vi "Update Step UI Values.vi"(9 "Array":string[][](array[string]), 10 "State cluster":T1, 11 "ListBox in":refnum<vi>) -> (2 "index of element":i32, 3 "Sequence #":i32)   [LabVIEW 2015, in "Sequencer Module tests.lvlib"]
uses:
  module/execution/Sequencer State Cluster.ctl
  module/execution/Sequencer State Enum.ctl
  classes/Step/Execution/StepState.ctl
  classes/Step/Execution/Step Status.ctl
  classes/Step/Execution/Step Flow Control.ctl
  Sequencer Module tests.lvlib
  module/execution/Sequencer Module runtime.lvclass
  classes/Step/Execution/Step.lvclass
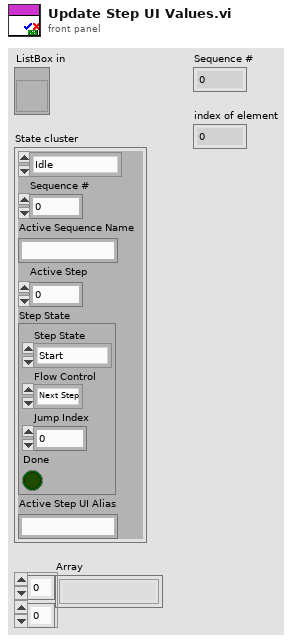
[diagram p1: front panel]
types:
  T1 = typedef "Sequencer Module runtime.lvclass/Sequencer State Cluster.ctl" = cluster{"Sequencer State":T2, "Sequence #":i32, "Active Sequence Name":string, "Active Step":i32, "Step State":T3, "Active Step UI Alias":string}
  T2 = typedef "Sequencer Module runtime.lvclass/Sequencer State Enum.ctl" = enum16{"Idle", "Paused", "Start Sequence", "Run Sequence", "CleanUp Sequence", "Generate Report"}
  T3 = typedef "Step.lvclass/StepState.ctl" = cluster{"Step State":T4, "Flow Control":T5, "Jump Index":i32, "Done":bool}
  T4 = typedef "Step.lvclass/Step Status.ctl" = enum16{"Start", "Passed", "Failed", "Error", "Done", "Terminated", "Skipped", "Running"}
  T5 = typedef "Step.lvclass/Step Flow Control.ctl" = enum16{"Next Step", "Jump"}
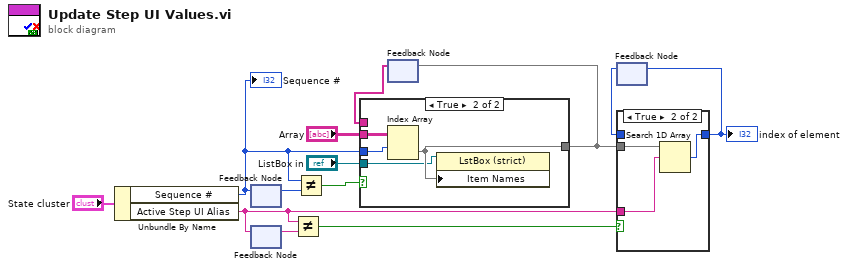
[diagram p0: block diagram]
diagram:
  n1 = Unbundle By Name("State cluster") -> ("Sequence #"=w6:i32, "Active Step UI Alias"=w11:string)
  "Sequence #" <- w6
  n2 = feedback #1() -> (w3:i32)  [unwired: 1 in]
  n3 = feedback-in #1(w6) -> ()
  n4 = feedback #2() -> (w8:string)  [unwired: 1 in]
  n5 = feedback-in #2(w11) -> ()
  n6 = Not Equal?(x=w11, y=w8) -> (x != y?=w9:bool)
  n7 = Not Equal?(x=w6, y=w3) -> (x != y?=w5:bool)
  n8 = feedback #3() -> (w7:string[])  [unwired: 1 in]
  n9 = case shown="True" w5 {
    tunnel: "Array" -> [_ w18]
    tunnel: w6 -> [_ w17]
    tunnel: [w14 w16] -> w10
    tunnel: w7 -> [w14 _]
    tunnel: "ListBox in" -> [_ w15]
    frame False {
    }
    frame True {
      n10 = Index Array(array=w18, index (row)=w17) -> (element=w16:string[])  [unwired: 1 in]
      n11 = property on="Property Node" class="LstBox (strict)"(reference=w15, "Item Names"=w16) -> ()  [unwired: 1 in, 2 out]
    }
  }
  n12 = feedback-in #3(w10) -> ()
  n13 = feedback #4() -> (w13:i32)  [unwired: 1 in]
  n14 = case shown="True" w9 {
    tunnel: w10 -> [_ w22]
    tunnel: w11 -> [_ w21]
    tunnel: [w19 w20] -> w12
    tunnel: w13 -> [w19 _]
    frame False {
    }
    frame True {
      n15 = Search 1D Array(1D array=w22, element=w21) -> (index of element=w20:i32)  [unwired: 1 in]
    }
  }
  "index of element" <- w12
  n16 = feedback-in #4(w12) -> ()
